vi "set integration time.vi"(8 "error in (no error)":errorcluster, 11 "LineCCD in":refnum<class "LineCCD.lvclass">) -> (0 "error out":errorcluster, 3 "LineCCD out":refnum<class "LineCCD.lvclass">)   [LabVIEW 2012, in "LineCCD.lvclass"]
uses:
  LineCCD.lvclass
  LineCCD.lvclass/LineCCD.ctl
  <instrlib>/ALPHALAS CCD S Series/ALPHALAS CCD S Series.lvlib
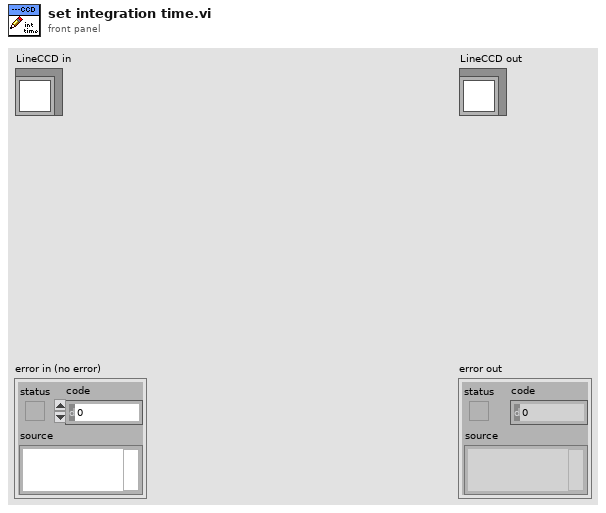
[diagram p1: front panel]
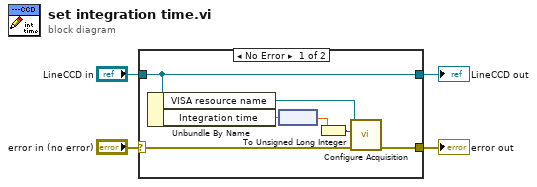
[diagram p0: block diagram]
diagram:
  n1 = case shown="No Error" "error in (no error)" {
    selector: "error in (no error)" -> [w9 w13]
    tunnel: [w8 w13] -> w3
    tunnel: [w11 w12] -> w1
    tunnel: "LineCCD in" -> [w11 w12]
    frame No Error {
      n2 = Unbundle By Name(w11) -> ("VISA resource name"=w10:refnum<visa-resource-name>, "Integration time"=w6:dbl[unit])
      n3 = node(w6) -> (w5:dbl)
      n4 = To Unsigned Long Integer(number=w5) -> (unsigned 32bit integer=w7:u32)
      n5 = call <instrlib>:"Configure Acquisition.vi"("error in (no error)"=w9, "Integration Time (5000 µs)"=w7, "VISA resource name"=w10) -> ("error out"=w8:errorcluster)  [unwired: 7 in, 1 out]
    }
    frame Error {
    }
  }
  "error out" <- w3
  "LineCCD out" <- w1
